vi "Update DOs Values.vi"(8 "error in":errorcluster, 11 "DOs Values":bool[](array[boolean])) -> (0 "error out":errorcluster)   [LabVIEW 2021, in "RT Interpreter.lvlib"]
uses:
  RT Interpreter.lvlib
  Libraries/UDP Comms/UDP Message--cluster.ctl
  Libraries/UDP Comms/UDP Comms.lvlib
panel:
  out "AOs Values":sgl[](array[numeric])
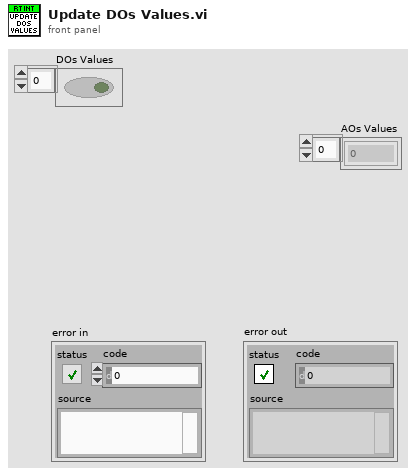
[diagram p1: front panel]
types:
  T1 = typedef "UDP Comms.lvlib/UDP Message--cluster.ctl" = cluster{"Command":string, "Data":variant}
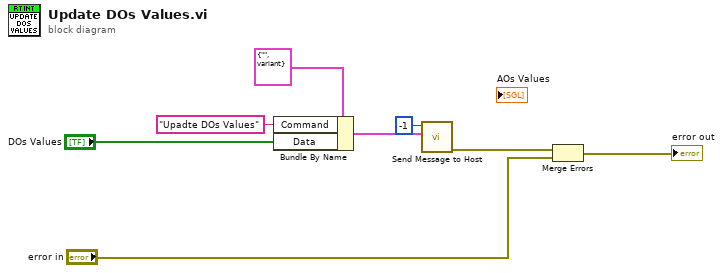
[diagram p0: block diagram]
diagram:
  n1 = Bundle By Name(cluster=T1 {"Command"="", "Data"=variant} ("UDP Message"), "Command"="Upadte DOs Values", "Data"="DOs Values") -> (w7:T1)
  n2 = call "Send Message to Host.vi"("UDP Message"=w7, "Module ID"=-1) -> ("error out"=w5:errorcluster)  [unwired: 9 in]
  n3 = Merge Errors(w5, "error in") -> (→"error out":errorcluster)
